vi "Fetch Backlog (U64).vi"(8 "error in":errorcluster, 11 "FPGA Session":T1) -> (0 "error out":errorcluster, 1 "Fetch Backlog":u32, 3 "FPGA Session":T1)   [LabVIEW 2011, in "FlexRIO Host Library (User).lvlib"]
uses:
  <userlib>/FlexRIO Host Library/FlexRIO Host Library (User).lvlib
  <userlib>/FlexRIO Host Library/FlexRIO Host API/Session/FPGA Session Ref.ctl
  <vilib>/Utility/error.llb/Error Cluster From Error Code.vi
  <vilib>/rvi/errors/niLvFpgaAdjustHostInterfaceError.vi
  <vilib>/rvi/interface/nirviMethod/nirviMethod.xnode
  OCT Reference Design/FPGA Bitfiles/OCTDigitizer_FPGABoard_AcquireDatawithout DRAM.lvbitx
  <vilib>/FPGAPlugInAG/PXIe-7965R/niLvFpga_ReadFifo_PXIe-7965R.vi
  <vilib>/rvi/errors/niLvFpgaMergeErrorWithErrorCode.vi
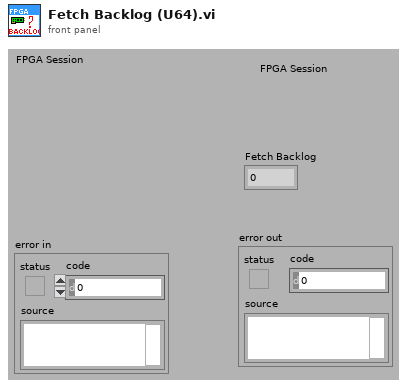
[diagram p1: front panel]
types:
  T1 = typedef "FlexRIO Host Library (User).lvlib/FPGA Session Ref.ctl" = refnum<k20>
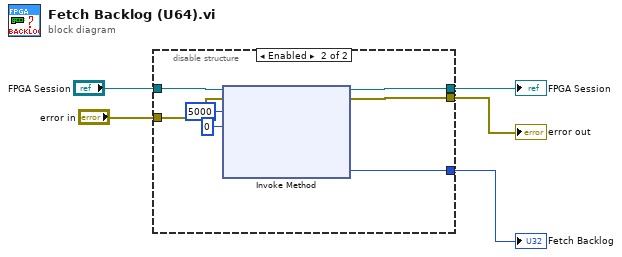
[diagram p0: block diagram]
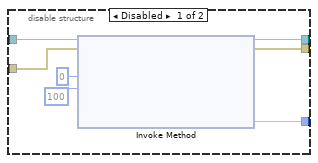
[diagram p2: hidden frame]
diagram:
  n1 = disable-structure shown="Enabled" {
    disable-tunnel: "FPGA Session" -> [w12 w19]
    disable-tunnel: "error in" -> [w11 w18]
    disable-tunnel: [w8 w13] -> w3
    disable-tunnel: [w7 w16] -> w2
    disable-tunnel: [w6 w17] -> w1
    frame Disabled {
      n2 = xnode "Invoke Method"("FPGA VI Reference In"=w12, "error in"=w11, "Number of Elements"=u32 0, "Timeout (ms)"=100) -> ("FPGA VI Reference Out"=w6:T1, "error out"=w7:errorcluster, "Elements Remaining"=w8)  [unwired: 1 out]
    }
    frame Enabled {
      n3 = xnode "Invoke Method"("FPGA VI Reference In"=w19, "error in"=w18, "Number of Elements"=u32 0, "Timeout (ms)"=5000) -> ("FPGA VI Reference Out"=w17:T1, "error out"=w16:errorcluster, "Elements Remaining"=w13:u32)  [unwired: 1 out]
    }
  }
  "Fetch Backlog" <- w3
  "error out" <- w2
  "FPGA Session" <- w1
